vi "Word_Chart_Font.vi"(0 "axes in":refnum<k7>, 1 "number format":string, 5 "type":i32(ring)=1 items=["xlCategory"=1, "xlSeriesAxis"=3, "xlValue"=2], 11 "error in":errorcluster, 12 "axis font":T1={"font style"="", "bold"=FALSE, "italic"=FALSE, "underline"=FALSE, "size"=10.0, "color"=4278190080} {"size" format="%.2f"}, 13 "title":string) -> (4 "axes out":refnum<k7>, 15 "error out":errorcluster)   [LabVIEW 2020, in "NI_ReportGenerationToolkit.lvlib"]
uses:
  <vilib>/addons/_office/NI_ReportGenerationToolkit.lvlib
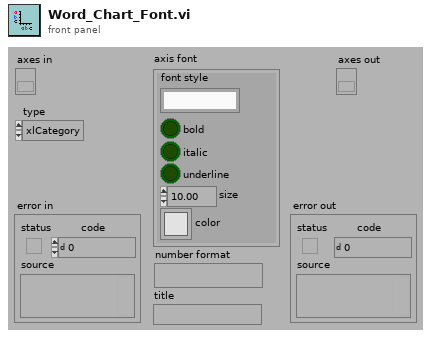
[diagram p1: front panel]
types:
  T1 = cluster{"font style":string, "bold":bool, "italic":bool, "underline":bool, "size":sgl, "color":u32}
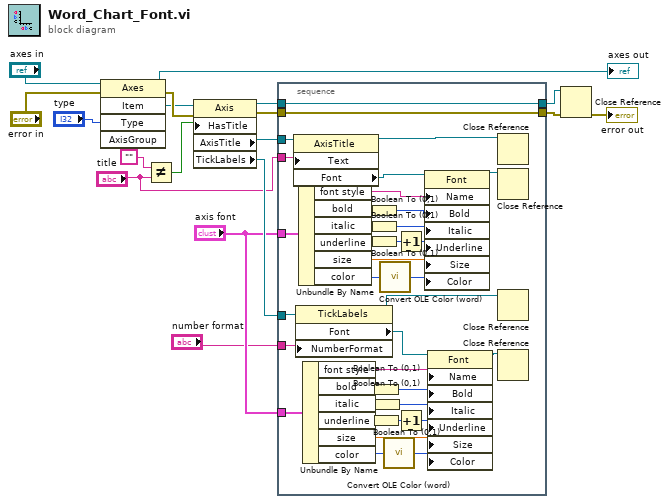
[diagram p0: block diagram]
diagram:
  n1 = invoke class="Axes" method="Item"(reference="axes in", error in="error in", "Type"="type") -> (reference out=→"axes out":refnum<k7>, error out=w16:errorcluster, "Item"=w14:refnum<k7>)  [unwired: 2 in, 2 out]
  n2 = Not Equal?(x="", y="title") -> (x != y?=w7:bool)
  n3 = property class="Axis"(reference=w14, error in=w16, "HasTitle"=w7) -> (reference out=w12:refnum<k7>, error out=w10:errorcluster, "AxisTitle"=w6:refnum<k7>, "TickLabels"=w5:refnum<k7>)
  n4 = stacked-sequence {
    tunnel: w12 -> [w53]
    tunnel: [w53] -> w11
    tunnel: w10 -> [w54]
    tunnel: [w54] -> w9
    tunnel: w6 -> [w52]
    tunnel: w5 -> [w50]
    tunnel: "axis font" -> [w48]
    tunnel: "axis font" -> [w47]
    tunnel: "title" -> [w29]
    tunnel: "number format" -> [w21]
    frame #0 {
      n5 = property class="AxisTitle"(reference=w52, "Text"=w29) -> (reference out=w28:refnum<k7>, "Font"=w51:refnum<k7>)  [unwired: 1 in, 1 out]
      n6 = property class="TickLabels"(reference=w50, "NumberFormat"=w21) -> (reference out=w26:refnum<k7>, "Font"=w49:refnum<k7>)  [unwired: 1 in, 1 out]
      n7 = Unbundle By Name(w48) -> ("font style"=w43:string, "bold"=w46:bool, "italic"=w45:bool, "underline"=w44:bool, "size"=w39:sgl, "color"=w38:u32)
      n8 = Unbundle By Name(w47) -> ("font style"=w37:string, "bold"=w36:bool, "italic"=w34:bool, "underline"=w32:bool, "size"=w31:sgl, "color"=w30:u32)
      n9 = Boolean To (0,1)(Boolean=w46) -> (0, 1=w42:i16)
      n10 = Boolean To (0,1)(Boolean=w45) -> (0, 1=w41:i16)
      n11 = Boolean To (0,1)(Boolean=w44) -> (0, 1=w40:i16)
      n12 = Boolean To (0,1)(Boolean=w36) -> (0, 1=w35:i16)
      n13 = Boolean To (0,1)(Boolean=w32) -> (0, 1=w24:i16)
      n14 = Boolean To (0,1)(Boolean=w34) -> (0, 1=w33:i16)
      n15 = call <vilib>:"Convert OLE Color (word).vi"("color in"=w38) -> ("color out"=w19:u32)
      n16 = call <vilib>:"Convert OLE Color (word).vi"("color in"=w30) -> ("color out"=w20:u32)
      n17 = Increment(x=w40) -> (x+1=w23:i16)
      n18 = Increment(x=w24) -> (x+1=w22:i16)
      n19 = property class="Font"(reference=w51, "Name"=w43, "Bold"=w42, "Italic"=w41, "Underline"=w23, "Size"=w39, "Color"=w19) -> (reference out=w27:refnum<k7>)  [unwired: 1 in, 1 out]
      n20 = property class="Font"(reference=w49, "Name"=w37, "Bold"=w35, "Italic"=w33, "Underline"=w22, "Size"=w31, "Color"=w20) -> (reference out=w25:refnum<k7>)  [unwired: 1 in, 1 out]
      n21 = Close Reference(reference=w28) -> ()  [unwired: 1 in, 1 out]
      n22 = Close Reference(reference=w27) -> ()  [unwired: 1 in, 1 out]
      n23 = Close Reference(reference=w26) -> ()  [unwired: 1 in, 1 out]
      n24 = Close Reference(reference=w25) -> ()  [unwired: 1 in, 1 out]
    }
  }
  n25 = Close Reference(reference=w11, error in (no error)=w9) -> (error out=→"error out":errorcluster)
